vi "未命名 3.vi"(0 "Image In":T2, 1 "Image Dst":T2, 7 "error in":errorcluster) -> (20 "Image Out":T2, 27 "error out":errorcluster)   [LabVIEW 2017]
doc: "Creates, edits, and runs vision algorithms using NI Vision Assistant.\n\nWhen you place this Express VI on the block diagram, NI Vision Assistant launches. Create an algorithm using the Vision Assistant processing functions. After you create an algorithm, you can select the controls and indicators that you want to be able to programmatically set in LabVIEW. Double-click the Vision Assistant Express VI to edit the algorithm."
uses:
  <vilib>/vision/Image Controls.llb/IMAQ Image.ctl
  <vilib>/vision/Pattern Matching.llb/IMAQ Curve Parameters.ctl
  <vilib>/vision/Pattern Matching.llb/IMAQ Match Range Setting.ctl
panel:
  in  "Reference System":T1={"Origin"={"X"=454.4994, "Y"=479.48618}, "Angle (deg)"=0.00021803747, "Axis Reference"=0} {"Axis Reference" items=["Direct", "Indirect"]}
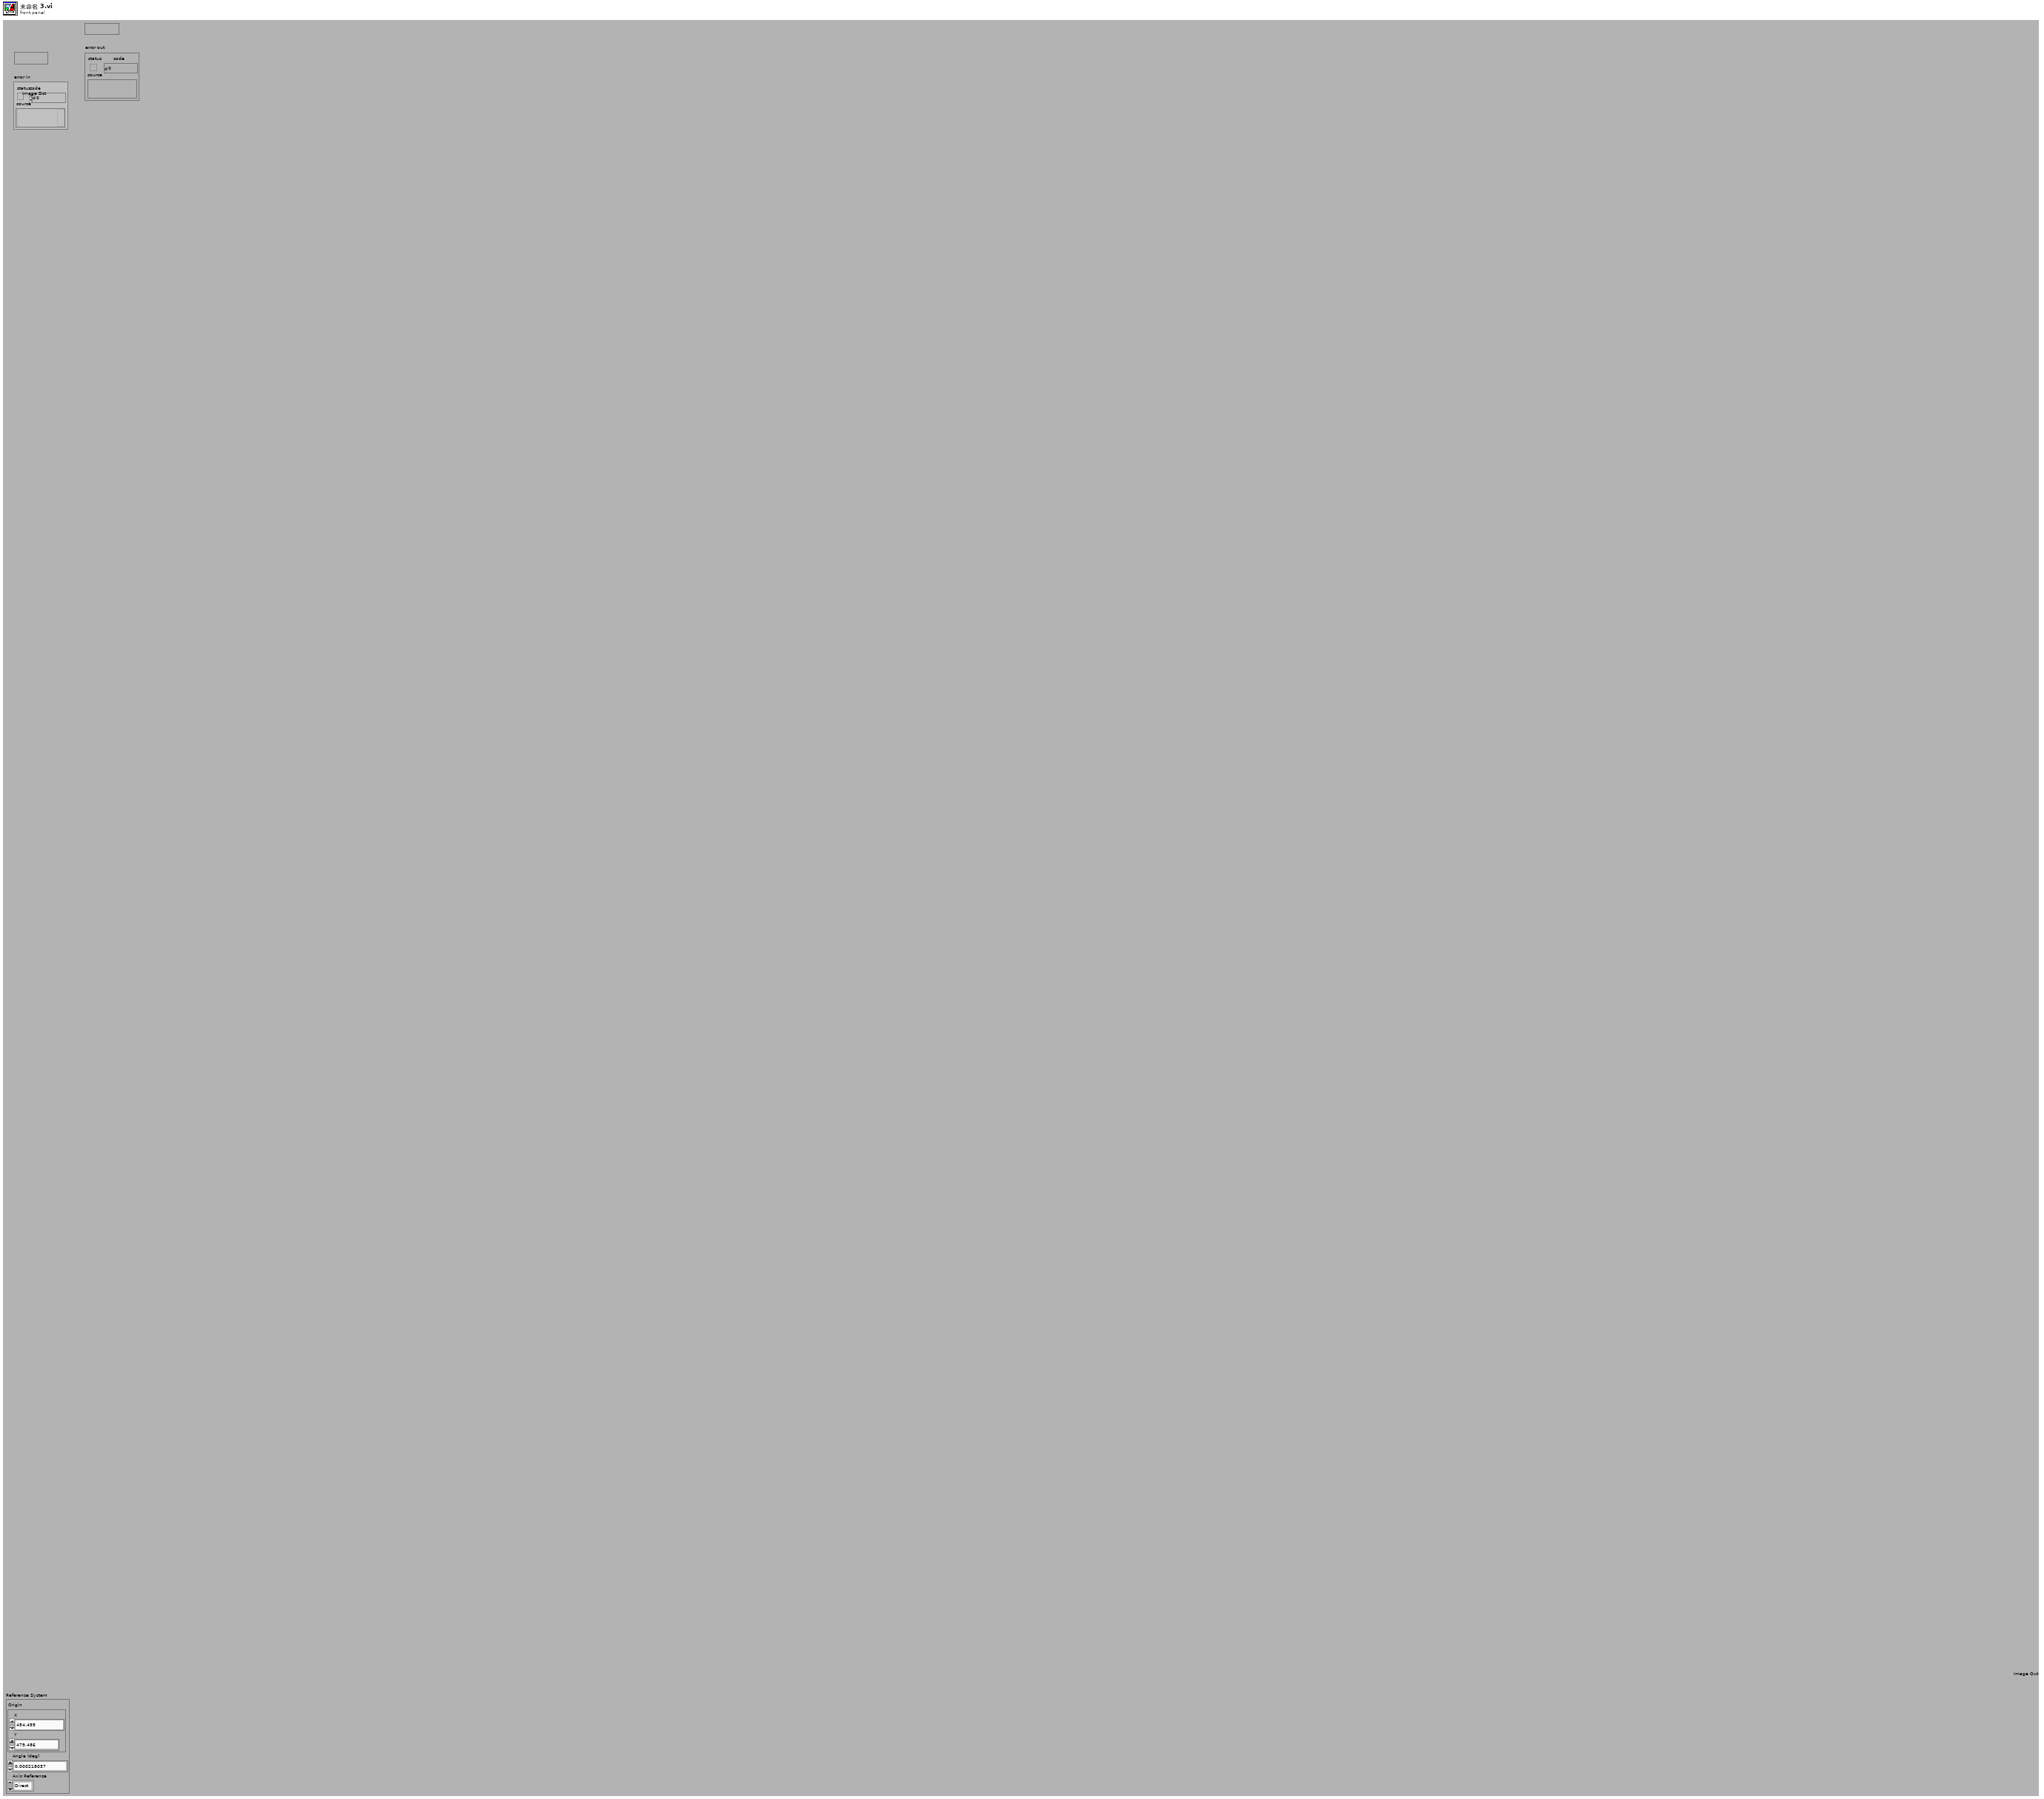
[diagram p1: front panel]
types:
  T1 = cluster{"Origin":cluster{"X":sgl, "Y":sgl}, "Angle (deg)":sgl, "Axis Reference":u32}
  T2 = typedef "IMAQ Image.ctl" = refnum<image>
  T3 = enum16{"Reset", "Update Coordinate System", "Get Coordinate System"}
  T4 = enum16{"Horizontal Motion", "Vertical Motion", "Horizontal and Vertical Motion", "Horizontal, Vertical and Angular Motion"}
  T5 = typedef "IMAQ Curve Parameters.ctl" = cluster{"Extraction Mode":u32, "Edge Threshold":i32, "Edge Filter Size":u32, "Min Length":i32, "Row Search Step Size":i32, "Col Search Step Size":i32, "Max Endpoint Gap":i32, "Closed":bool, "Subpixel":bool}
  T6 = typedef "IMAQ Match Range Setting.ctl" = cluster{"Match Constraints":u32, "Min":dbl, "Max":dbl}
  T7 = cluster{"Curve Parameters":T5, "Match Mode":cluster{"Rotation":bool, "Scale":bool, "Occlusion":bool, "Reserved 1":bool, "Reserved 2":bool, "Reserved 3":bool}, "Range Settings":T6[], "Number of Matches":i32, "Minimum Match Score":sgl, "SubPixel Accuracy":bool, "Adv. Geometric Match Options 2":cluster{"Setup Data Item":u16, "Item Value":dbl}[]}
  T8 = cluster{"Global Rectangle":i32[], "Contours":cluster{"ID":enum32{"External", "Internal"}, "Type":u32, "Coordinates":i32[]}[]}
  T9 = typedef "Image Type" = u32
  T10 = typedef "IMAQ GM Match Report.ctl" = cluster{"Position":cluster{"x":sgl, "y":sgl}, "Angle":sgl, "Scale":sgl, "Score":sgl, "Bounding Box":cluster{"x":sgl, "y":sgl}[], "Contrast Reversed":bool, "Occlusion %":sgl, "Template Target Curve Score":sgl, "Target Template Curve Score":sgl, "Correlation Score":sgl}
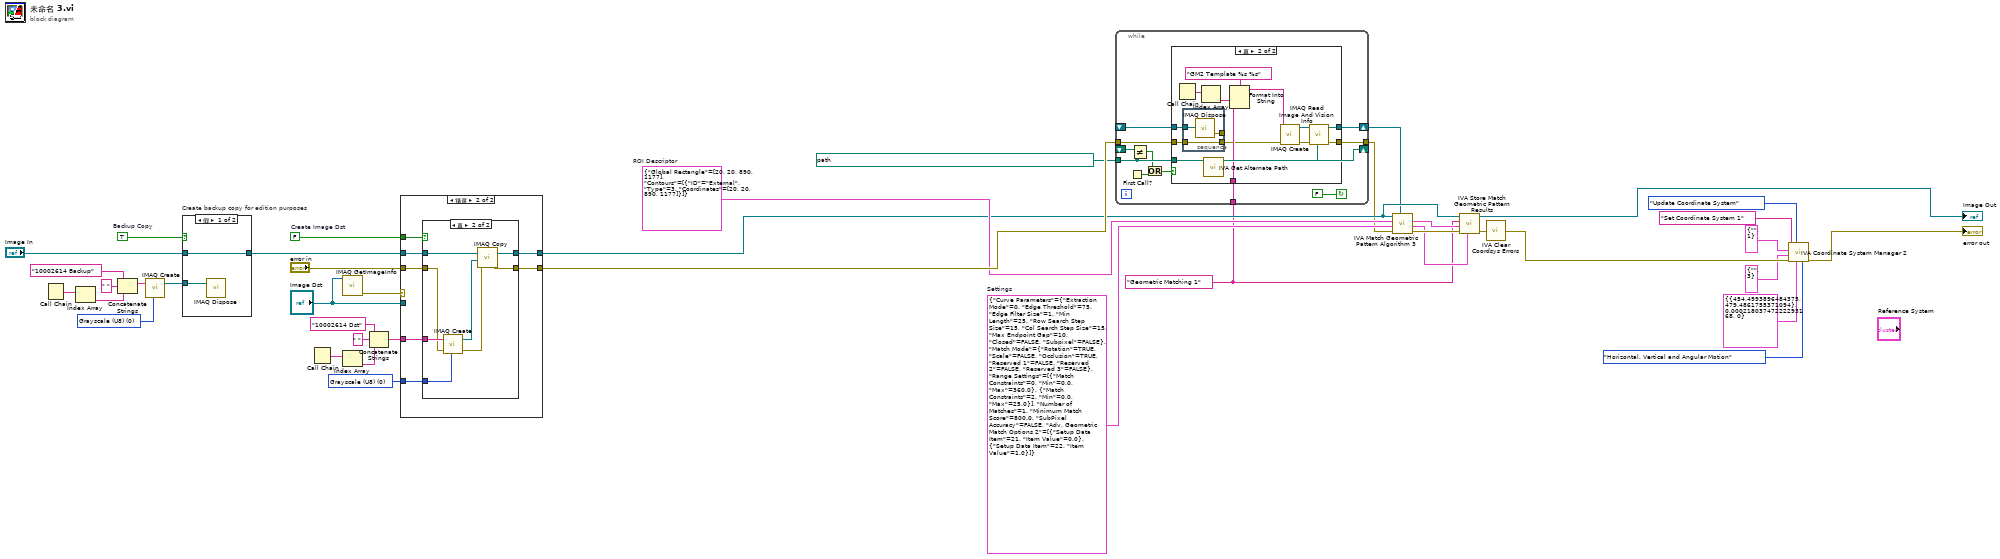
[diagram p0: block diagram]
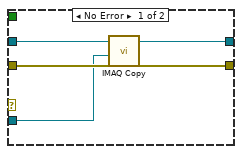
[diagram p3: hidden frame]
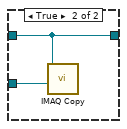
[diagram p5: hidden frame]
diagram:
  w14 = T7 {"Curve Parameters"={"Extraction Mode"=0, "Edge Threshold"=75, "Edge Filter Size"=1, "Min Length"=25, "Row Search Step Size"=15, "Col Search Step Size"=15, "Max Endpoint Gap"=10, "Closed"=FALSE, "Subpixel"=FALSE}, "Match Mode"={"Rotation"=TRUE, "Scale"=FALSE, "Occlusion"=TRUE, "Reserved 1"=FALSE, "Reserved 2"=FALSE, "Reserved 3"=FALSE}, "Range Settings"=[{"Match Constraints"=0, "Min"=0.0, "Max"=360.0}, {"Match Constraints"=2, "Min"=0.0, "Max"=25.0}], "Number of Matches"=1, "Minimum Match Score"=800.0, "SubPixel Accuracy"=FALSE, "Adv. Geometric Match Options 2"=[{"Setup Data Item"=21, "Item Value"=0.0}, {"Setup Data Item"=22, "Item Value"=1.0}]}  # Settings
  w13 = "Geometric Matching 1" ("Step Name")
  w19 = T8 {"Global Rectangle"=[20, 20, 890, 1177], "Contours"=[{"ID"=enum."External", "Type"=3, "Coordinates"=[20, 20, 890, 1177]}]}  # ROI Descriptor
  w21 = T9 0 items=["Grayscale (U8)", "Grayscale (I16)", "Grayscale (SGL)", "Complex (CSG)", "RGB (U32)", "HSL (U32)", "RGB (U64)", "Grayscale (U16)"] ("Image Dst Type")
  w22 = T9 0 items=["Grayscale (U8)", "Grayscale (I16)", "Grayscale (SGL)", "Complex (CSG)", "RGB (U32)", "HSL (U32)", "RGB (U64)", "Grayscale (U16)"] ("Image Type")
  w41 = TRUE  # Backup Copy
  w34 = FALSE  # Create Image Dst
  n1 = Call Chain() -> (call chain=w28:string[])
  n2 = Index Array(array=w28) -> (element=w27:string)  [unwired: 1 in]
  n3 = Concatenate Strings("10002614 Backup" ("Backup Image Name"), " ", w27) -> (w24:string)
  n4 = call "IMAQ Create"("Image Name"=w24, "Image Type"=w22) -> ("New Image"=w23:T2)  [unwired: 2 in, 2 out]
  n5 = case "Create backup copy for edition purposes" shown="假" w41 {
    tunnel: [w43 w45] -> w37
    tunnel: "Image In" -> [w43 w45]
    tunnel: w23 -> [w42 w44]
    frame False {
      n6 = call "IMAQ Dispose"("Image"=w42) -> ()  [unwired: 2 in, 4 out]
    }
    frame True {
      n7 = call "IMAQ Copy"("Image Dst"=w44, "Image Src"=w45) -> ()  [unwired: 1 in, 5 out]
    }
  }
  n8 = Call Chain() -> (call chain=w33:string[])
  n9 = call "IMAQ GetImageInfo"("Image"="Image Dst") -> ("error out"=w39:errorcluster)  [unwired: 1 in, 9 out]
  n10 = Index Array(array=w33) -> (element=w31:string)  [unwired: 1 in]
  n11 = Concatenate Strings("10002614 Dst" ("Image Dst Name"), " ", w31) -> (w29:string)
  n12 = case "条件结构" shown="错误" w39 {
    tunnel: [w50 w54] -> w15
    tunnel: [w49 w53] -> w35
    tunnel: w37 -> [w48 w55]
    tunnel: "error in" -> [w47 w51]
    tunnel: "Image Dst" -> [w46 _]
    tunnel: w29 -> [_ w57]
    tunnel: w21 -> [_ w56]
    tunnel: w34 -> [_ w52]
    frame No Error {
      n13 = call "IMAQ Copy"("error in (no error)"=w47, "Image Dst"=w46, "Image Src"=w48) -> ("error out"=w49:errorcluster, "Image Dst Out"=w50:T2)  [unwired: 3 out]
    }
    frame Error {
      n14 = case "条件结构" shown="真" w52 {
        tunnel: w57 -> [_ w67]
        tunnel: w56 -> [_ w66]
        tunnel: w55 -> [w59 w64]
        tunnel: [w59 w63] -> w54
        tunnel: [w58 w62] -> w53
        tunnel: w51 -> [w58 w60]
        frame False {
        }
        frame True {
          n15 = call "IMAQ Create"("Image Name"=w67, "Image Type"=w66, "error in (no error)"=w60) -> ("New Image"=w65:T2, "error out"=w61:errorcluster)  [unwired: 1 in, 1 out]
          n16 = call "IMAQ Copy"("error in (no error)"=w61, "Image Dst"=w65, "Image Src"=w64) -> ("error out"=w62:errorcluster, "Image Dst Out"=w63:T2)  [unwired: 3 out]
        }
      }
    }
  }
  n17 = while {
    shift-right: [w78] -> w11
    shift-left: _ -> [w77]
    tunnel: [w75] -> w12
    tunnel: w35 -> [w74]
    tunnel: path "D:/Inspect System/Source Code/Template Program/字符检测定位模板.png" ("Template File Path") -> [w71]
    tunnel: w13 -> [w73]
    shift-right: [w71] -> _
    shift-left: _ -> [w72]
    stop <- FALSE continue-if-true
    n18 = First Call?() -> (First Call?: T/F=w70:bool)
    n19 = Not Equal?(x=w72, y=w71) -> (x != y?=w69:bool)
    n20 = Or(x=w69, y=w70) -> (x .or. y?=w68:bool)
    n21 = case "条件结构" shown="真" w68 {
      tunnel: [w80 w92] -> w78
      tunnel: w77 -> [w80 w84]
      tunnel: [w79 w89] -> w75
      tunnel: w74 -> [w79 w85]
      tunnel: w73 -> [_ w86]
      tunnel: w71 -> [_ w83]
      frame False {
      }
      frame True {
        n22 = Call Chain() -> (call chain=w88:string[])
        n23 = stacked-sequence "层叠式顺序结构" {
          tunnel: w85 -> [w97]
          tunnel: w84 -> [w96]
          tunnel: [w97] -> w81
          tunnel: [w95] -> _
          frame #0 {
            n24 = call "IMAQ Dispose"("Image"=w96) -> ("error out"=w95:errorcluster)  [unwired: 2 in, 3 out]
          }
        }
        n25 = Index Array(array=w88) -> (element=w87:string)  [unwired: 1 in]
        n26 = call <vilib>:"IVA Get Alternate Path.vi"("Path In"=w83) -> ("Path Out"=w82:path)  [unwired: 10 out]
        n27 = Format Into String(format string="GM2 Template %s %s" ("Image Name"), w87, w86) -> (resulting string=w94:string)  [unwired: 2 in, 1 out]
        n28 = call "IMAQ Create"("Image Name"=w94, "error in (no error)"=w81) -> ("New Image"=w91:T2, "error out"=w90:errorcluster)  [unwired: 2 in, 1 out]
        n29 = call "IMAQ Read Image And Vision Info"("File Path"=w82, "error in (no error)"=w90, "Image"=w91) -> ("error out"=w89:errorcluster, "Image Out"=w92:T2)  [unwired: 1 in, 6 out]
      }
    }
  }
  n30 = call <vilib>:"IVA Match Geometric Pattern Algorithm 3.vi"("Template"=w11, "error in (no error)"=w12, "Settings"=w14, "ROI Descriptor"=w19, "Image"=w15) -> ("error out"=w18:errorcluster, "Calibrated Matches"=w16:T10[], "Matches"=w17:T10[])  [unwired: 4 out]
  n31 = call <vilib>:"IVA Store Match Geometric Pattern Results.vi"("Calibrated Matches"=w16, "error in (no error)"=w18, "Matches"=w17, "Step Name"=w13, "Image in"=w15) -> ("error out"=w10:errorcluster, "Image dup"=→"Image Out":T2)  [unwired: 5 out]
  n32 = call <vilib>:"IVA Clear Coordsys Errors.vi"("error in (no error)"=w10) -> ("error out"=w9:errorcluster)  [unwired: 10 in]
  n33 = call <vilib>:"IVA Coordinate System Manager 2.vi"("Mode"=T4."Horizontal, Vertical and Angular Motion", "Reference System"=T1 {"Origin"={"X"=454.4994, "Y"=479.48618}, "Angle (deg)"=0.00021803747, "Axis Reference"=0}, "Function"=T3."Update Coordinate System", "error in (no error)"=w9, "Angle ID"=cluster{"GUID":string, "Index":i32} {"GUID"="", "Index"=3}, "Origin ID"=cluster{"GUID":string, "Index":i32} {"GUID"="", "Index"=1}, "Coordinate System Name"="Set Coordinate System 1") -> ("error out"=→"error out":errorcluster)  [unwired: 4 out]
